vi "Populate Footers From Document.vi"(8 "error in (no error)":errorcluster, 11 "xwpfDocument in":refnum<class "xwpfDocument.lvclass">) -> (0 "error out":errorcluster, 3 "xwpfDocument out":refnum<class "xwpfDocument.lvclass">)   [LabVIEW 2017, in "Word_Specific.lvlib" / "xwpfDocument.lvclass"]
uses:
  xwpfDocument.lvclass
  xwpfDocument.lvclass/xwpfDocument.ctl
  C:/Users/Neo/Desktop/Dev_Tools_BR/LabVIEW_NPOI/src/lib/NPOI 2.1.1/NPOI.OOXML.dll
  lib/NPOI 2.1.1/NPOI.OOXML.dll
  xwpfHeader_Footer/xwpfHeader_Footer.lvclass
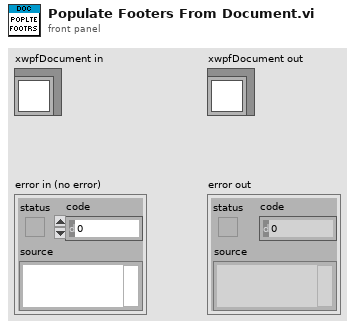
[diagram p1: front panel]
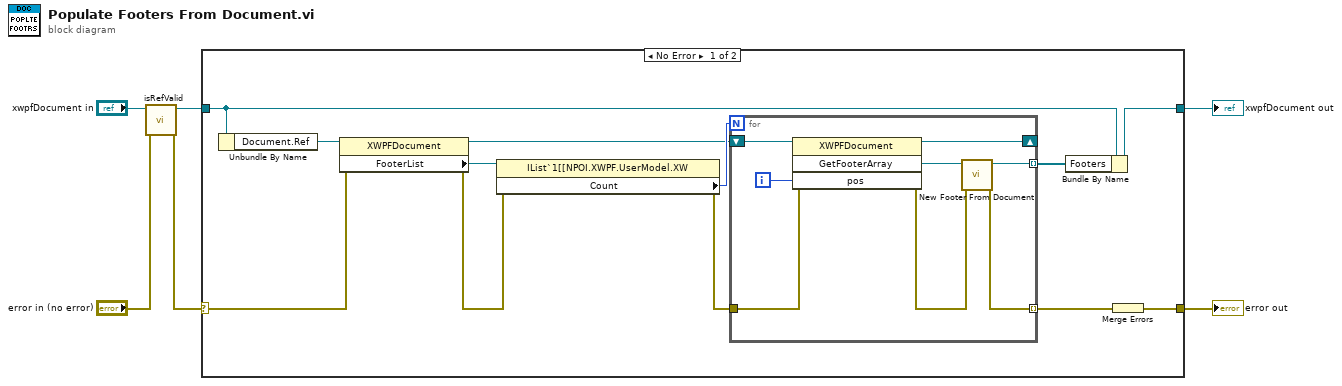
[diagram p0: block diagram]
diagram:
  n1 = call-dynamic "isRefValid.vi"("error in (no error)"="error in (no error)", "xwpfDocument in"="xwpfDocument in") -> ("error out"=w1:errorcluster, "xwpfDocument out"=w3:refnum<class "xwpfDocument.lvclass">)  [unwired: 8 in]
  n2 = case shown="No Error" w1 {
    selector: w1 -> [w14 w28]
    tunnel: [w7 w28] -> w6
    tunnel: [w10 w27] -> w4
    tunnel: w3 -> [w11 w27]
    frame No Error {
      n3 = Unbundle By Name(w11) -> ("Document.Ref"=w8:refnum<k24>)
      n4 = property class="XWPFDocument"(reference=w8, error in=w14) -> (reference out=w9:refnum<k24>, error out=w15:errorcluster, "FooterList"=w18:refnum<k24>)
      n5 = property class="IList`1[[NPOI.XWPF.UserModel.XW"(reference=w18, error in=w15) -> (error out=w16:errorcluster, "Count"=w17:i32)  [unwired: 1 out]
      n6 = for {
        N: w17 -> [_]
        shift-right: [w24] -> _
        shift-left: w9 -> [w26]
        tunnel: [w22] -> w12 mode=indexing
        tunnel: w16 -> [w23]
        tunnel: [w19] -> w13 mode=indexing
        i -> [w25]
        n7 = invoke class="XWPFDocument" method="GetFooterArray"(reference=w26, error in=w23, "pos"=w25) -> (reference out=w24:refnum<k24>, error out=w20:errorcluster, "GetFooterArray"=w21:refnum<k24>)  [unwired: 1 in, 1 out]
        n8 = call "New Footer From Document.vi"("error in (no error)"=w20, "Footer Ref"=w21) -> ("error out"=w19:errorcluster, "xwpfHeader out"=w22:refnum<class "xwpfHeader_Footer.lvclass">)  [unwired: 8 in]
      }
      n9 = Bundle By Name(cluster=w11, "Footers"=w12) -> (w10:refnum<class "xwpfDocument.lvclass">)
      n10 = Merge Errors(w13) -> (w7:errorcluster)
    }
    frame Error {
    }
  }
  "error out" <- w6
  "xwpfDocument out" <- w4
